vi "Cont Gen Voltage Wfm-Int Clk-Non Regeneration_Core.vi"() -> ()   [LabVIEW 2011]
doc: "I. Description:\nThis example demonstrates how to continuously output a waveform using an internal sample clock. The automatic regeneration of data has been disabled, so new data has to be provided throughout the duration of the continuous Analog Output operation. This allows the generation of any arbitrary frequency as this VI computes new data for each iteration of the loop, maintaining phase continuity of the signal.\n\nII. Instructions for Running:\n1. Select the Physical Channel to correspond to where your signal is output on the DAQ device.\n2. Enter the Minimum and Maximum Voltage range.\n3. Specify the desired Sample Clock Rate of the output Waveform. Higher sample clock rates will produce a smoother waveform.\n4. Manually specify the Analog Output buffer size, in number of samples. A larger buffer would help non-regenerative operations avoid errors due to occasional high CPU load. \nNote: \nThe Analog Output buffer has to be at least as big as the amount of data being written to the board per iteration. The recommended buffer size would be at least twice the amount of data being written to the board per iteration.\n5. Enter the Waveform Information. See the documentation of the Basic Function Generator SubVI for information on each parameter.\n\nIII. Block Diagram Steps:\n1. Create an Analog Output Voltage channel.\n2. Configure the task to prohibit the automatic regeneration of data.\n3. Call the DAQmx (Sample Clock) VI to set the sample clock rate. Additionally, set the sample mode to Continuous.\n4. Read the actual sample clock rate (eventually coerced depending on the hardware used). \n5. Compute the desired waveform, using the buffer size and the actual update rate. This VI keeps track of the phase of the waveform to ensure that the generated signal is continuous.\n6. Write the waveform to the output buffer. \n7a. Call the Start VI. This is only needed when the loop is executed for the first time.\n7b. Do nothing.\n8. Loop continuously until user presses the Stop button. Every iteration computes and writes a new waveform to the buffer.\n9. Call the Clear Task VI to clear the Task.\n10. Use the popup dialog box to display an error or warning if any.\n\nIV. I/O Connections Overview:\nMake sure your signal output terminal matches the Physical Channel I/O Control. For further connection information, refer to your hardware reference manual."
uses:
  <vilib>/Utility/error.llb/DialogType.ctl
  <vilib>/DAQmx/write.llb/DAQmx Write (Analog 1D Wfm NChan NSamp).vi
  <vilib>/DAQmx/create/channels.llb/DAQmx Create Channel (AO-Voltage-Basic).vi
  <vilib>/DAQmx/configure/timing.llb/DAQmx Timing (Sample Clock).vi
  <vilib>/DAQmx/miscellaneous.llb/DAQmx Fill In Error Info.vi
  <vilib>/measure/NI_MABase.lvlib
  Program Files (x86)/National Instruments/LabVIEW 2011/resource/objmgr/daqmx.rc
panel:
  in  "offset 2":dbl format="%0.2p"
  in  "offset":dbl=7.0 format="%0.2p"
  in  "Amplitude 2":dbl=5.0 caption="Amplitude" format="%0.2p"
  in  "Frequency 2":dbl=5.0 caption="Frequency" format="%.2f"
  in  "Waveform Type 2":T1(ring) caption="Waveform Type"
  in  "#s":u32=5020 caption="Size (Samples)"
  out "Actual Sample\nClock Rate":dbl=5000.0 format="%.2f"
  in  "Sample Clock Rate":dbl=5000.0 format="%0.2f"
  in  "Waveform Type":T1(ring)=enum."Square Wave"
  in  "Frequency":dbl=10.0 format="%.2f"
  in  "Amplitude":dbl=2.5 format="%0.2p"
  out "Waveform Graph":waveform(dbl)[](graph)=[{"t0"=timestamp(539.148 s since 1904-01-01), "dt"=0.0002, "Y"=array[5020 elements]}, {"t0"=timestamp(539.148 s since 1904-01-01), "dt"=0.0002, "Y"=array[5020 elements]}, {"t0"=timestamp(539.148 s since 1904-01-01), "dt"=0.0002, "Y"=array[5020 elements]}, {"t0"=timestamp(539.148 s since 1904-01-01), "dt"=0.0002, "Y"=array[5020 elements]}, {"t0"=timestamp(539.148 s since 1904-01-01), "dt"=0.0002, "Y"=array[5020 elements]}, {"t0"=timestamp(539.148 s since 1904-01-01), "dt"=0.0002, "Y"=array[5020 elements]}, {"t0"=timestamp(539.148 s since 1904-01-01), "dt"=0.0002, "Y"=array[5020 elements]}, {"t0"=timestamp(539.148 s since 1904-01-01), "dt"=0.0002, "Y"=array[5020 elements]}, {"t0"=timestamp(539.148 s since 1904-01-01), "dt"=0.0002, "Y"=array[5020 elements]}, {"t0"=timestamp(539.148 s since 1904-01-01), "dt"=0.0002, "Y"=array[5020 elements]}, {"t0"=timestamp(539.148 s since 1904-01-01), "dt"=0.0002, "Y"=array[5020 elements]}] caption="Output Waveform"
  in  "Physical Channels":tag="Dev2/ao0:10"
  in  "Minimum Value":dbl=-10.0 format="%0.2f"
  in  "Maximum Value":dbl=10.0 format="%0.2f"
  in  "stop":bool
  # "For instructions, select Help>>Show Context Help"
  # "Channel Parameters"
  # "Timing Parameters"
  # "Buffer Parameters"
  # "Waveform Information"
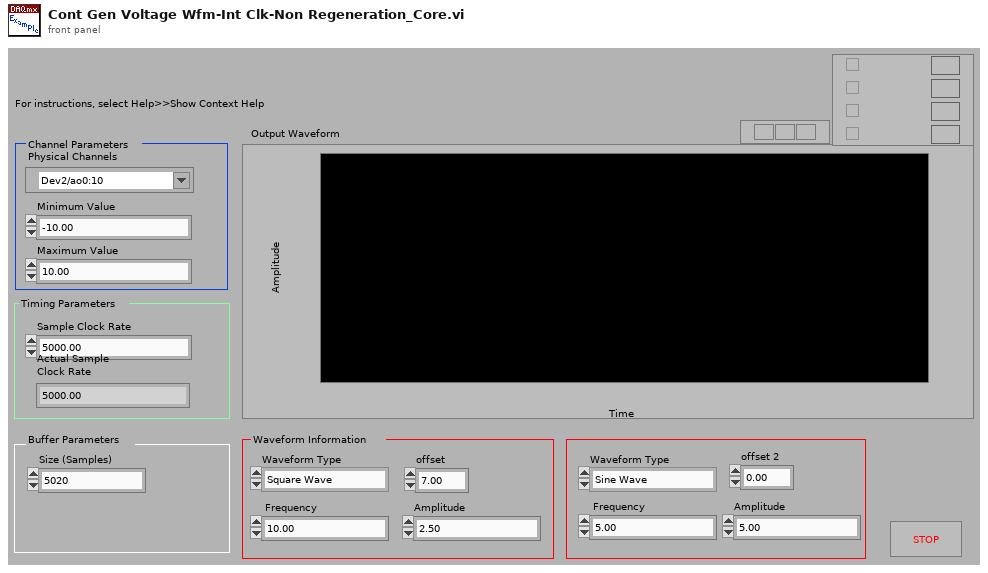
[diagram p1: front panel]
types:
  T1 = enum16{"Sine Wave", "Triangle Wave", "Square Wave", "Sawtooth Wave"}
  T2 = typedef "DialogType.ctl" = u16
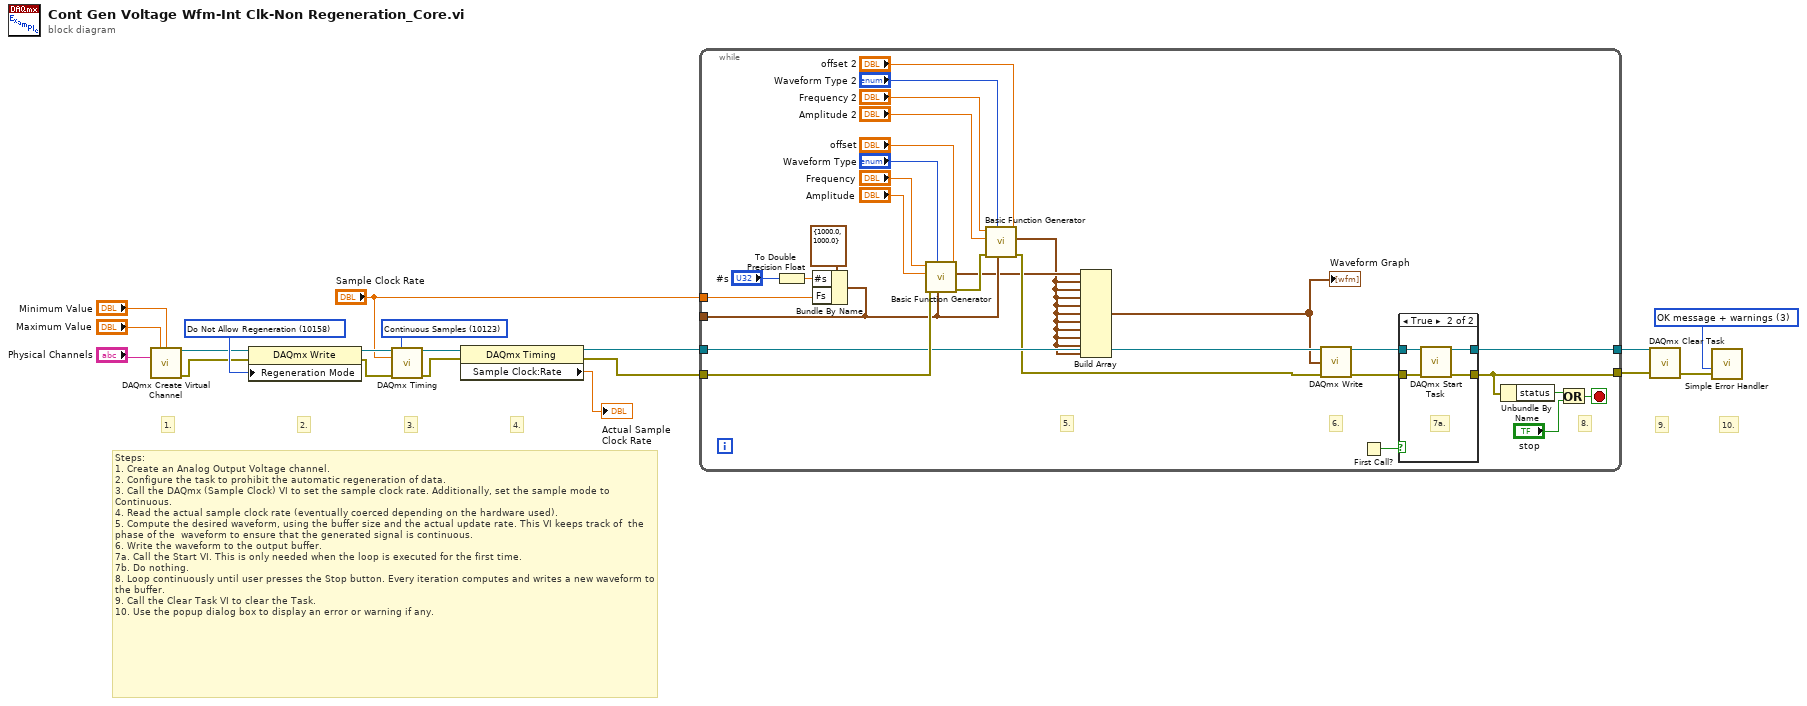
[diagram p0: block diagram]
diagram:
  w8 = 10158 items=["Allow Regeneration"=10097, "Do Not Allow Regeneration"=10158] ("RegenMode")
  w14 = T2 3 items=["no dialog", "OK message", "continue or stop message", "OK message + warnings", "continue/stop + warnings"] ("type of dialog (OK msg:1)")
  w18 = 10123 items=["Finite Samples"=10178, "Continuous Samples"=10123] ("sample mode")
  # "4."
  # "3."
  # "Steps:\n1. Create an Analog Output Voltage channel.\n2. Configure the task to prohibit the automatic regeneration of data.\n3. Call the DAQmx (Sample Clock) VI to set the sample clock rate. Additionally, set the sample mode to Continuous.\n4. Read the actual sample clock rate (eventually coerced depending on the hardware used).\n5. Compute the desired waveform, using the buffer size and the actual update rate. This VI keeps track of  the phase of the  waveform to ensure that the generated signal is continuous.\n6. Write the waveform to the output buffer. \n7a. Call the Start VI. This is only needed when the loop is executed for the first time.\n7b. Do nothing.\n8. Loop continuously until user presses the Stop button. Every iteration computes and writes a new waveform to the buffer.\n9. Call the Clear Task VI to clear the Task.\n10. Use the popup dialog box to display an error or warning if any."
  # "10."
  # "9."
  # "2."
  # "1."
  n1 = call-poly <vilib>:"DAQmx Create Virtual Channel.vi"("maximum value"="Maximum Value", "minimum value"="Minimum Value", "physical channels"="Physical Channels") -> ("task out"=w7:refnum<k21>, "error out"=w6:errorcluster)  [unwired: 6 in, 5 out]
  n2 = property class="DAQmx Write"(reference=w7, error in=w6, "Regeneration Mode"=w8) -> (reference out=w3:refnum<k21>, error out=w2:errorcluster)
  n3 = call-poly <vilib>:"DAQmx Timing.vi"("task/channels in"=w3, "sample mode"=w18, "rate"="Sample Clock Rate", "error in"=w2) -> ("task out"=w11:refnum<k21>, "error out"=w10:errorcluster)  [unwired: 3 in, 7 out]
  n4 = property class="DAQmx Timing"(reference=w11, error in=w10) -> (reference out=w5:refnum<k21>, error out=w4:errorcluster, "Sample Clock:Rate"=→"Actual Sample\nClock Rate":dbl)
  n5 = while {
    tunnel: w5 -> [w43]
    tunnel: [w39] -> w13
    tunnel: w4 -> [w44]
    tunnel: [w40] -> w12
    tunnel: [w23] -> _
    tunnel: "Sample Clock Rate" -> [w22]
    stop <- w47 stop-if-true
    # "8."
    # "6."
    # "5."
    n6 = To Double Precision Float(number="#s") -> (double precision float=w26:dbl)
    n7 = Bundle By Name(cluster=cluster{"Fs":dbl, "#s":dbl} {"Fs"=1000.0, "#s"=1000.0} ("sampling info"), "#s"=w26, "Fs"=w22) -> (w23:cluster{"Fs":dbl, "#s":dbl})
    n8 = call <vilib>:"Basic Function Generator.vi"("offset"="offset", "sampling info"=w23, "signal type"="Waveform Type", "error in (no error)"=w44, "amplitude"="Amplitude", "frequency"="Frequency") -> ("error out"=w28:errorcluster, "signal out"=w21:waveform(dbl))  [unwired: 3 in, 1 out]
    n9 = call <vilib>:"Basic Function Generator.vi"("offset"="offset 2", "sampling info"=w23, "signal type"="Waveform Type 2", "error in (no error)"=w28, "amplitude"="Amplitude 2", "frequency"="Frequency 2") -> ("error out"=w27:errorcluster, "signal out"=w20:waveform(dbl))  [unwired: 3 in, 1 out]
    n10 = Build Array(w21, w20, w20, w20, w20, w20, w20, w20, w20, w20, w20) -> (w31:waveform(dbl)[])
    "Waveform Graph" <- w31
    n11 = call-poly <vilib>:"DAQmx Write.vi"("task/channels in"=w43, "data"=w31, "error in"=w27) -> ("task out"=w42:refnum<k21>, "error out"=w41:errorcluster)  [unwired: 1 in, 10 out]
    n12 = First Call?() -> (First Call?: T/F=w38:bool)
    n13 = case shown="True" w38 {
      tunnel: w42 -> [w49 w53]
      tunnel: w41 -> [w48 w52]
      tunnel: [w48 w51] -> w40
      tunnel: [w49 w50] -> w39
      frame False {
        # "7b."
      }
      frame True {
        # "7a."
        n14 = call <vilib>:"DAQmx Start Task.vi"("task/channels in"=w53, "error in"=w52) -> ("task out"=w50:refnum<k21>, "error out"=w51:errorcluster)  [unwired: 12 out]
      }
    }
    n15 = Unbundle By Name(w40) -> ("status"=w46:bool)
    n16 = Or(x=w46, y="stop") -> (x .or. y?=w47:bool)
  }
  n17 = call <vilib>:"DAQmx Clear Task.vi"("task in"=w13, "error in"=w12) -> ("error out"=w19:errorcluster)  [unwired: 13 out]
  n18 = call <vilib>:"Simple Error Handler.vi"("type of dialog (OK msg:1)"=w14, "error in (no error)"=w19) -> ()  [unwired: 8 out]
